vi "GetCurveRefParam.vi"(8 "错误输入（无错误）":errorcluster) -> (0 "错误输出":errorcluster)   [LabVIEW 2014]
uses:
  ZXUTConfigMgr.dll
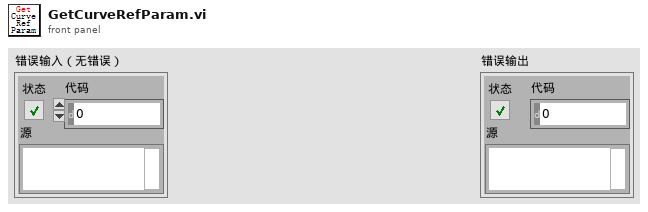
[diagram p1: front panel]
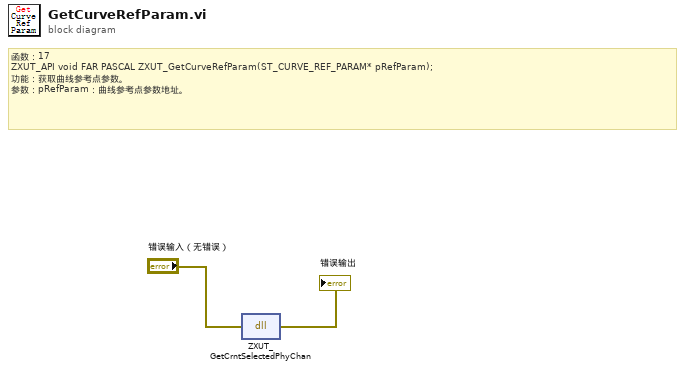
[diagram p0: block diagram]
diagram:
  # "函数：17\nZXUT_API void\tFAR PASCAL ZXUT_GetCurveRefParam(ST_CURVE_REF_PARAM* pRefParam);\n功能：获取曲线参考点参数。\n参数：pRefParam：曲线参考点参数地址。"
  n1 = dll-call lib="PTH2eabs D软件超声实时监测软件ZXUTAppDemo(华南理工V02.00)X86DllZXUTConfigMgr.dll" fn="ZXUT_GetCrntSelectedPhyChan"(error in="错误输入（无错误）") -> (error out=→"错误输出":errorcluster)  [unwired: 3 in, 1 out]
